vi "Read Screen Head.vi"(8 "error in":errorcluster, 11 "OWON SDS1022.lvclass":refnum<class "OWON SDS1022.lvclass">) -> (0 "error out":errorcluster, 2 "Head <JSON>":string, 3 "OWON SDS1022.lvclass 2":refnum<class "OWON SDS1022.lvclass">)   [LabVIEW 2023, in "OWON SDS1022.lvclass"]
uses:
  OWON SDS1022.lvclass
  OWON SDS1022.lvclass/OWON SDS1022.ctl
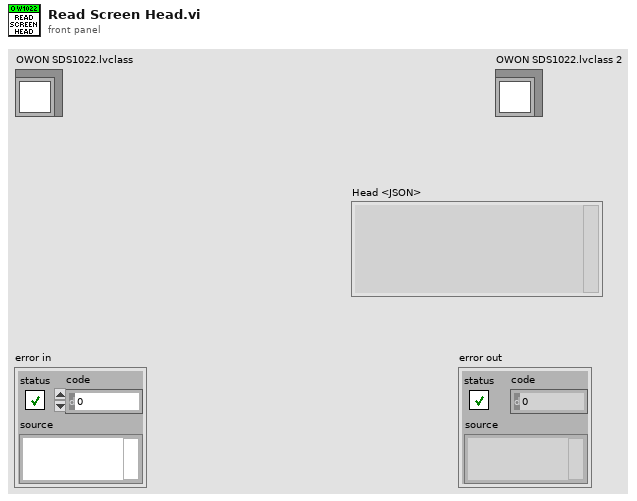
[diagram p1: front panel]
types:
  T1 = enum16{"big-endian, network order", "native, host order", "little-endian"}
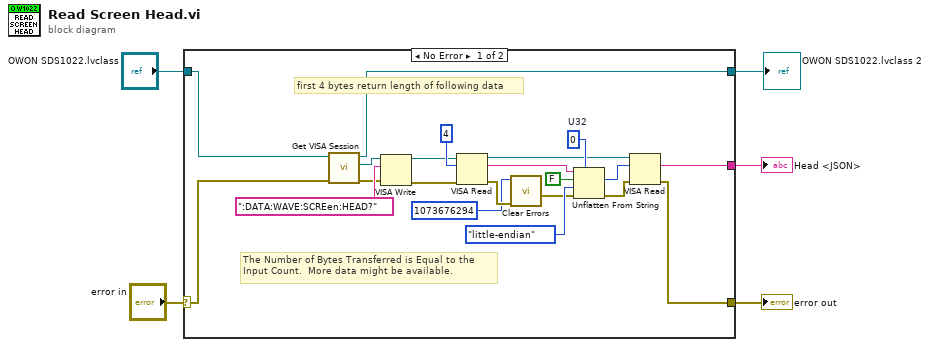
[diagram p0: block diagram]
diagram:
  n1 = case shown="No Error" "error in" {
    selector: "error in" -> [w9 w28]
    tunnel: [w13 w28] -> w4
    tunnel: [w12 _] -> w3
    tunnel: "OWON SDS1022.lvclass" -> [w10 w27]
    tunnel: [w7 w27] -> w1
    frame No Error {
      w21 = u32 0  # U32
      # "The Number of Bytes Transferred is Equal to the \nInput Count.  More data might be available."
      # "first 4 bytes return length of following data"
      n2 = call-dynamic "Get VISA Session.vi"("error in"=w9, "Scope VISA in"=w10) -> ("error out"=w6:errorcluster, "VISA session"=w8:refnum<visa-resource-name>, "Scope VISA out"=w7:refnum<class "OWON SDS1022.lvclass">)  [unwired: 7 in]
      n3 = VISA Write(VISA resource name=w8, write buffer=":DATA:WAVE:SCREen:HEAD?", error in (no error)=w6) -> (VISA resource name out=w11:refnum<visa-resource-name>, error out=w23:errorcluster)  [unwired: 1 out]
      n4 = VISA Read(VISA resource name=w11, byte count=u32 4, error in (no error)=w23) -> (VISA resource name out=w16:refnum<visa-resource-name>, read buffer=w17:string, error out=w24:errorcluster)  [unwired: 1 out]
      n5 = call <vilib>:"Clear Errors.vi"("error in (no error)"=w24, "specific error code to clear (0: all)"=1073676294) -> ("error out"=w18:errorcluster)  [unwired: 4 in, 1 out]
      n6 = Unflatten From String(type=w21, binary string=w17, data includes array or string size? (T)=FALSE, byte order (0:big-endian, network order)=T1."little-endian", error in (no error)=w18) -> (value=w14:u32, error out=w15:errorcluster)  [unwired: 1 out]
      n7 = VISA Read(VISA resource name=w16, byte count=w14, error in (no error)=w15) -> (read buffer=w12:string, error out=w13:errorcluster)  [unwired: 2 out]
    }
    frame Error {
    }
  }
  "error out" <- w4
  "Head <JSON>" <- w3
  "OWON SDS1022.lvclass 2" <- w1
